vi "Get Producer Values.vi"(8 "error in":errorcluster, 11 "Chiller Cluster.lvclass":refnum<class "Chiller Cluster.lvclass">) -> (0 "error out":errorcluster, 1 "Producer Ch":T1(array[cluster]), 2 "Producer Control":T2, 3 "Chiller Cluster.lvclass out":refnum<class "Chiller Cluster.lvclass">)   [LabVIEW 2023, in "Chiller Cluster.lvclass"]
uses:
  Chiller Cluster.lvclass
  Chiller Cluster.lvclass/Chiller Cluster.ctl
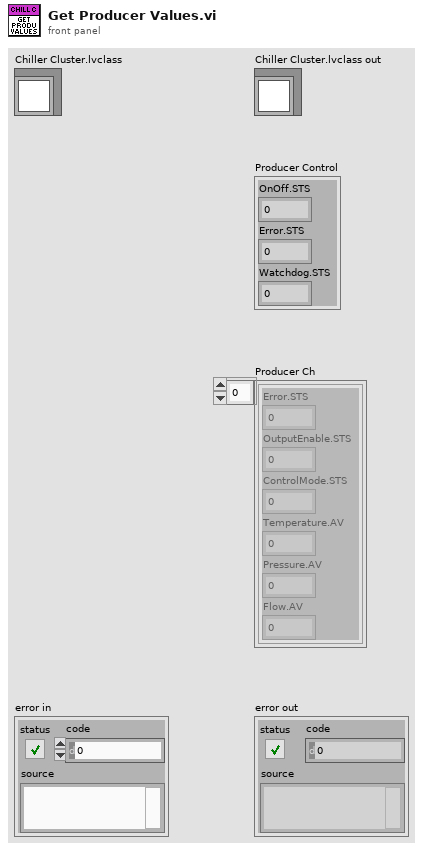
[diagram p1: front panel]
types:
  T1 = cluster{"Error.STS":i32, "OutputEnable.STS":i32, "ControlMode.STS":u16, "Temperature.AV":dbl, "Pressure.AV":dbl, "Flow.AV":dbl}[]
  T2 = cluster{"OnOff.STS":i32, "Error.STS":i32, "Watchdog.STS":i32}
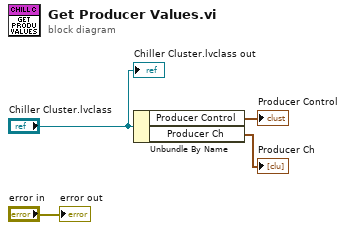
[diagram p0: block diagram]
diagram:
  n1 = Unbundle By Name("Chiller Cluster.lvclass") -> ("Producer Control"=→"Producer Control":T2, "Producer Ch"=→"Producer Ch":T1)
  "error out" <- "error in"
  "Chiller Cluster.lvclass out" <- "Chiller Cluster.lvclass"
